vi "string array selection.vi"(5 "regular expression":string, 7 "selection":T1(ring), 11 "files":cluster{"String":string, "Boolean":bool}[](array[cluster])) -> (2 "wild card?":bool, 3 "files 2":cluster{"String":string, "Boolean":bool}[](array[cluster]))   [LabVIEW 2025]
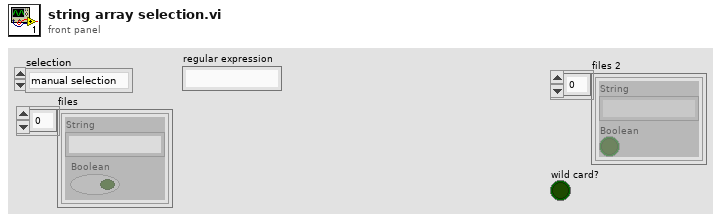
[diagram p1: front panel]
types:
  T1 = enum16{"manual selection", "select all", "unselect all", "inverse selection", "use wild card"}
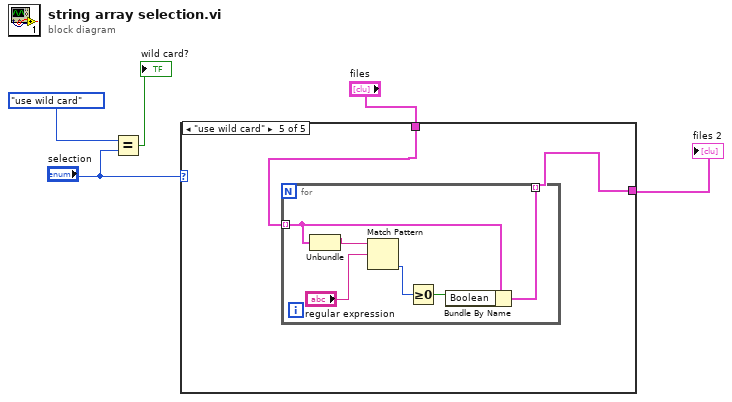
[diagram p0: block diagram]
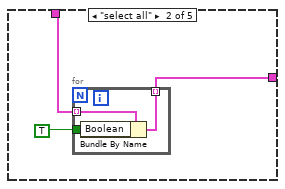
[diagram p3: hidden frame]
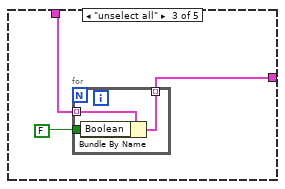
[diagram p4: hidden frame]
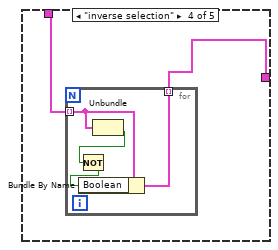
[diagram p5: hidden frame]
diagram:
  n1 = Equal?(x=T1."use wild card" ("selection"), y="selection") -> (x = y?=→"wild card?":bool)
  n2 = case shown="\"use wild card\"" "selection" {
    tunnel: "files" -> [w6 w9 w15 w20 w25]
    tunnel: [w6 w8 w14 w19 w26] -> w4
    frame "manual selection", Default {
    }
    frame "select all" {
      n3 = for {
        tunnel: w9 -> [w11] mode=indexing
        tunnel: [w12] -> w8 mode=indexing
        tunnel: TRUE -> [w10]
        n4 = Bundle By Name(cluster=w11, "Boolean"=w10) -> (w12:cluster{"String":string, "Boolean":bool})
      }
    }
    frame "unselect all" {
      n5 = for {
        tunnel: w15 -> [w17] mode=indexing
        tunnel: [w18] -> w14 mode=indexing
        tunnel: FALSE -> [w16]
        n6 = Bundle By Name(cluster=w17, "Boolean"=w16) -> (w18:cluster{"String":string, "Boolean":bool})
      }
    }
    frame "inverse selection" {
      n7 = for {
        tunnel: w20 -> [w23] mode=indexing
        tunnel: [w24] -> w19 mode=indexing
        n8 = Unbundle(w23) -> ("Boolean"=w22:bool)  [unwired: 1 out]
        n9 = Not(x=w22) -> (.not. x?=w21:bool)
        n10 = Bundle By Name(cluster=w23, "Boolean"=w21) -> (w24:cluster{"String":string, "Boolean":bool})
      }
    }
    frame "use wild card" {
      n11 = for {
        tunnel: w25 -> [w31] mode=indexing
        tunnel: [w32] -> w26 mode=indexing
        n12 = Unbundle(w31) -> ("String"=w30:string)  [unwired: 1 out]
        n13 = Match Pattern(string=w30, regular expression="regular expression") -> (offset past match=w28:i32)  [unwired: 1 in, 3 out]
        n14 = Greater Or Equal To 0?(x=w28) -> (x >= 0?=w27:bool)
        n15 = Bundle By Name(cluster=w31, "Boolean"=w27) -> (w32:cluster{"String":string, "Boolean":bool})
      }
    }
  }
  "files 2" <- w4
